vi "GetComboboxReference.vi"(8 "error in":errorcluster, 11 "Combobox in":refnum<class "Combobox.lvclass">) -> (0 "error out":errorcluster, 1 "Combobox reference":refnum<vi>, 3 "Combobox out":refnum<class "Combobox.lvclass">)   [LabVIEW 2014, in "Combobox.lvclass"]
uses:
  Combobox.lvclass
  Generic/Generic.lvclass
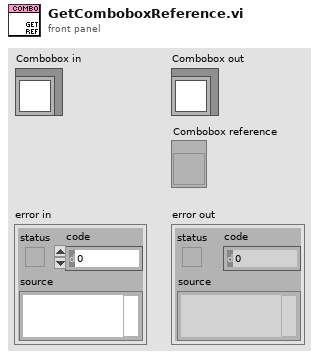
[diagram p1: front panel]
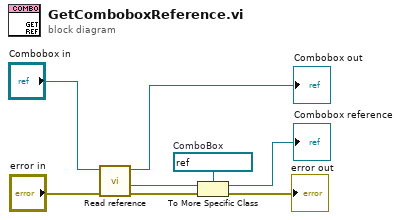
[diagram p0: block diagram]
diagram:
  w6 = refnum<vi> refnum  # ComboBox
  n1 = call "Read reference.vi"("error in"="error in", "GObject in"="Combobox in") -> ("error out"=w7:errorcluster, "reference"=w8:refnum<vi>, "GObject out"=→"Combobox out":refnum<class "Combobox.lvclass">)  [unwired: 5 in]
  n2 = To More Specific Class(target class=w6, reference=w8, error in=w7) -> (specific class reference=→"Combobox reference":refnum<vi>, error out=→"error out":errorcluster)
